vi "CAN.Initialize.vi"(8 "error in (no error)":errorcluster, 11 "Diagnostics Basic Configuration":T5) -> (0 "error out":errorcluster, 3 "Diagnostics Configuration":T1={"Interface"="", "Baud Rate"=0, "Diagnostic Protocol"=enum."GMLAN", "Transport Protocol"=enum."ISO TP - Normal Mode", "Transmit ID"=0, "Receive ID"=0, "Transmit Extension"=0, "Receive Extension"=0, "Receive UUDT ID"=0, "Enable Stream"=TRUE, "VW TP Channel ID"=0, "Fill Frame"=FALSE, "Fill Byte"=255, "Termination"=FALSE, "LIN Cluster"="ADCS_LIN_database", "NAD"=1, "IO Mode"=0, "Max DLC"=8, "FD Baud Rate"=0, "Timeout"=0, "FD ISO Mode"=0, "DoIP Address"="", "DoIP Source Address"=3584, "DoIP Dynamic Port"=TRUE, "DoIP Version"=2} {"DoIP Version" items=["2010"=1, "2012"=2]; "DoIP Source Address" format="%.0x"; "FD ISO Mode" items=["ISO", "Non ISO", "ISO Legacy"]; "IO Mode" items=["CAN 2.0", "CAN FD", "CAN FD+BRS"]; "Fill Byte" format="%.0x"; "VW TP Channel ID" format="%.0x"; "Receive UUDT ID" format="%.0x"; "Receive Extension" format="%.0x"; "Transmit Extension" format="%.0x"; "Receive ID" format="%.0x"; "Transmit ID" format="%.0x"})   [LabVIEW 2024, in "Diagnostics Addon System Explorer.lvlib"]
uses:
  Diagnostics Addon System Explorer.lvlib
  Types/Addon.Initialize.ctl
  Addon Shared/Types/Protocol.ctl
  Addon Shared/Types/CAN.ctl
  Addon Shared/Types/CAN.Interface.ctl
  Addon Shared/Types/Transport.ctl
  Addon Shared/Diagnostics Addon Shared.lvlib
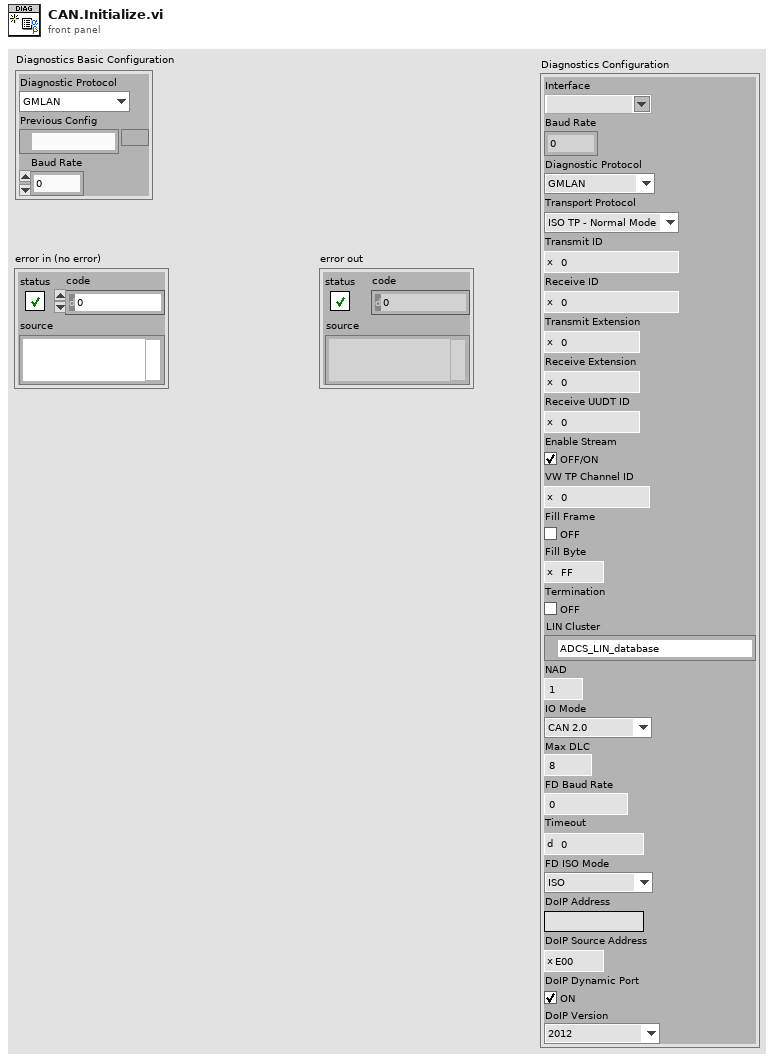
[diagram p1: front panel]
types:
  T1 = typedef "Diagnostics Addon Shared.lvlib/CAN.ctl" = cluster{"Interface":T2, "Baud Rate":u64, "Diagnostic Protocol":T3, "Transport Protocol":T4, "Transmit ID":u32, "Receive ID":u32, "Transmit Extension":u8, "Receive Extension":u8, "Receive UUDT ID":u32, "Enable Stream":bool, "VW TP Channel ID":u32, "Fill Frame":bool, "Fill Byte":u8, "Termination":bool, "LIN Cluster":refnum<k21>, "NAD":u8, "IO Mode":u32, "Max DLC":u16, "FD Baud Rate":u64, "Timeout":u32, "FD ISO Mode":u32, "DoIP Address":string, "DoIP Source Address":u16, "DoIP Dynamic Port":bool, "DoIP Version":u16}
  T2 = typedef "Diagnostics Addon Shared.lvlib/CAN.Interface.ctl" = string
  T3 = typedef "Diagnostics Addon Shared.lvlib/Protocol.ctl" = enum16{"GMLAN", "KWP-2000", "UDS", "User-Defined"}
  T4 = typedef "Diagnostics Addon Shared.lvlib/Transport.ctl" = enum16{"ISO TP - Normal Mode", "ISO TP - Mixed Mode", "VW TP 2.0", "Diagnostics on IP", "ISO TP LIN"}
  T5 = typedef "Diagnostics Addon System Explorer.lvlib/Addon.Initialize.ctl" = cluster{"Diagnostic Protocol":T3, "Previous Config":path, "Baud Rate":u32}
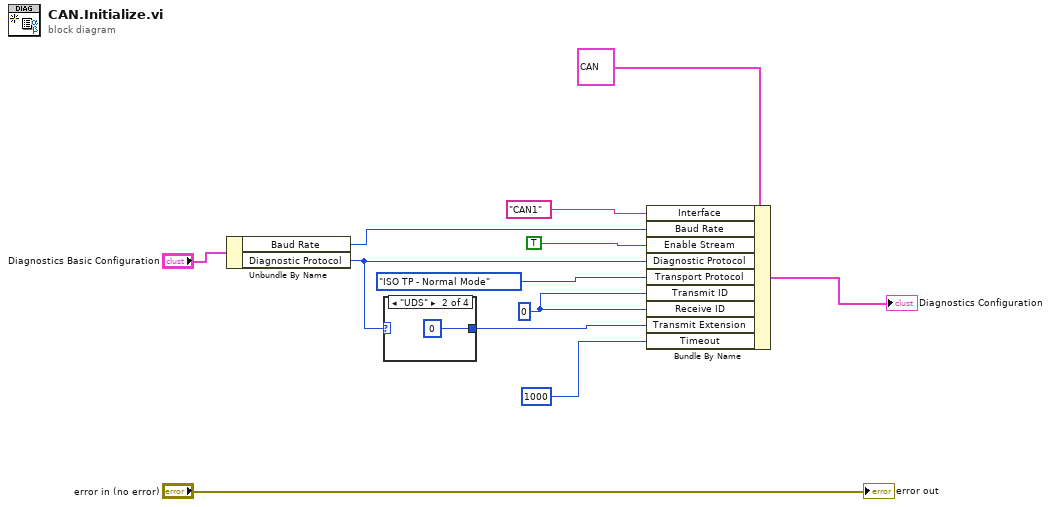
[diagram p0: block diagram]
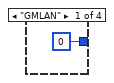
[diagram p2: hidden frame]
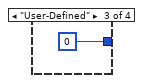
[diagram p3: hidden frame]
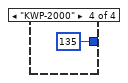
[diagram p4: hidden frame]
diagram:
  w9 = u32 0 ("Transmit ID")
  n1 = Unbundle By Name("Diagnostics Basic Configuration") -> ("Baud Rate"=w3:u32, "Diagnostic Protocol"=w11:T3)
  n2 = case shown="\"UDS\"" w11 {
    tunnel: [u8 0 ("Mode ID") u8 0 ("Mode ID") u8 0 ("Mode ID") u8 135 ("Mode ID")] -> w7
    frame "GMLAN" {
    }
    frame "UDS" {
    }
    frame "User-Defined" {
    }
    frame "KWP-2000" {
    }
  }
  n3 = Bundle By Name(cluster=T1 {"Interface"="", "Baud Rate"=0, "Diagnostic Protocol"=enum."GMLAN", "Transport Protocol"=enum."ISO TP - Normal Mode", "Transmit ID"=0, "Receive ID"=0, "Transmit Extension"=0, "Receive Extension"=0, "Receive UUDT ID"=0, "Enable Stream"=TRUE, "VW TP Channel ID"=0, "Fill Frame"=FALSE, "Fill Byte"=255, "Termination"=FALSE, "LIN Cluster"="ADCS_LIN_database", "NAD"=1, "IO Mode"=0, "Max DLC"=8, "FD Baud Rate"=0, "Timeout"=0, "FD ISO Mode"=0, "DoIP Address"="", "DoIP Source Address"=3584, "DoIP Dynamic Port"=TRUE, "DoIP Version"=2} ("Diagnostics Basic Configuraiton"), "Interface"="CAN1" ("Diagnostics Basic Configuraiton.CAN Interface"), "Baud Rate"=w3, "Enable Stream"=TRUE, "Diagnostic Protocol"=w11, "Transport Protocol"=Transport."ISO TP - Normal Mode", "Transmit ID"=w9, "Receive ID"=w9, "Transmit Extension"=w7, "Timeout"=u32 1000 ("Diagnostics Basic Configuraiton.Timeout")) -> (→"Diagnostics Configuration":T1)
  "error out" <- "error in (no error)"
